vi "exchange data.vi"(8 "error in":errorcluster, 9 "timeout in ms (0)":i32, 10 "data table in":T1, 11 "buffer exchange":T2) -> (0 "error out":errorcluster, 1 "exchange failed":bool, 2 "data table out":T1)   [LabVIEW 2013, in "tag bus buffer exchange.lvlib"]
uses:
  tag bus buffer exchange.lvlib
  buffer exchange.ctl
  buffer reference.ctl
  table/data table.ctl
  table/data table.lvlib
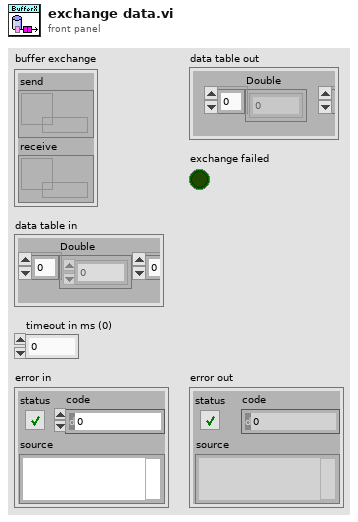
[diagram p1: front panel]
types:
  T1 = typedef "tag bus.lvlib/data table.lvlib/data table.ctl" = cluster{"Double":dbl[], "Single":sgl[], "I64":i64[], "I32":i32[], "I16":i16[], "I8":i8[], "U64":u64[], "U32":u32[], "U16":u16[], "U8":u8[], "Boolean":bool[], "String":string[], "Array of Double":cluster{"DBL Array":dbl[]}[], "Array of Single":cluster{"SGL Array":sgl[]}[], "Array of I64":cluster{"I64 Array":i64[]}[], "Array of I32":cluster{"I32 Array":i32[]}[], "Array of I16":cluster{"I16 Array":i16[]}[], "Array of I8":cluster{"I8 Array":i8[]}[], "Array of U64":cluster{"U64 Array":u64[]}[], "Array of U32":cluster{"U32 Array":u32[]}[], "Array of U16":cluster{"U16 Array":u16[]}[], "Array of U8":cluster{"U8 Array":u8[]}[], "Array of Boolean":cluster{"Boolean Array":bool[]}[], "Array of String":cluster{"String Array":string[]}[]}
  T2 = typedef "tag bus buffer exchange.lvlib/buffer exchange.ctl" = cluster{"send":refnum<k33>, "receive":refnum<k33>}
  T3 = typedef "tag bus buffer exchange.lvlib/buffer reference.ctl" = refnum<data-value>
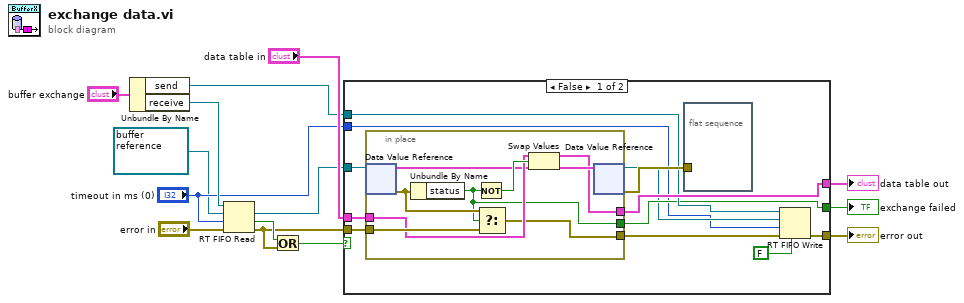
[diagram p0: block diagram]
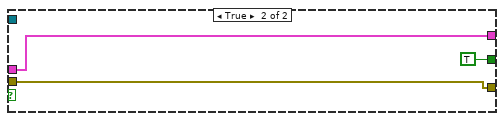
[diagram p2: hidden frame]
diagram:
  n1 = Unbundle By Name("buffer exchange") -> ("send"=w4:refnum<k33>, "receive"=w13:refnum<k33>)
  n2 = RT FIFO Read(0:w13, 1:T3 refnum ("Null DVR"), 2:"timeout in ms (0)", 3:"error in") -> (9:w5:T3, 10:w12:bool, 11:w10:errorcluster)  [unwired: 2 out]
  n3 = Or(x=w12, y=w10) -> (x .or. y?=w11:bool)
  n4 = case shown="False" w11 {
    tunnel: w10 -> [w25 w38]
    tunnel: [w21 w38] -> w9
    tunnel: [w18 TRUE] -> w8
    tunnel: [w22 w36] -> w7
    tunnel: "data table in" -> [w23 w36]
    tunnel: w5 -> [w26 _]
    tunnel: w4 -> [w19 _]
    tunnel: "timeout in ms (0)" -> [w16 _]
    frame False {
      n5 = in-place {
        in-place-border: w25 -> [w35]
        in-place-border: w23 -> [w33]
        in-place-border: [w30] -> w22
        in-place-border: [w29] -> w20
        in-place-border: [w27] -> w18
        n6 = in-place-dvr #1(w26) -> (w32:T1, w28:errorcluster)
        n7 = Unbundle By Name(w28) -> ("status"=w27:bool)
        n8 = Not(x=w27) -> (.not. x?=w34:bool)
        n9 = Select(t=w28, s=w27, f=w35) -> (s? t:f=w29:errorcluster)
        n10 = Swap Values(12:w33, 13:w34, 14:w32) -> (1:w30:T1, 3:w31:T1)
        n11 = in-place-dvr #1(w31) -> (w17:T3, w24:errorcluster)
      }
      n12 = flat-sequence {
        tunnel: w24 -> [_]
        frame #0 {
        }
      }
      n13 = RT FIFO Write(0:w19, 1:w17, 2:w16, 3:w20, 5:FALSE ("overwrite on timeout (T)")) -> (11:w21:errorcluster)  [unwired: 3 out]
    }
    frame True {
    }
  }
  "error out" <- w9
  "exchange failed" <- w8
  "data table out" <- w7
